vi "deleteScriptEvent.vi"(8 "error in (no error)":errorcluster, 10 "Enum":enum16{"Update_dt", "Update_Time"}(ring), 11 "ScriptEditorV2 in":refnum<class "ScriptEditorV2.lvclass">) -> (0 "error out":errorcluster, 3 "ScriptEditorV2 out":refnum<class "ScriptEditorV2.lvclass">)   [LabVIEW 2011, in "Views.lvlib" / "ScriptEditor.lvlib" / "ScriptEditorV2.lvclass"]
uses:
  ScriptEditorV2.lvclass
  ScriptEditorV2.lvclass/ScriptEditorV2.ctl
  Tools/Scripting/ScriptingEvent/ScriptEventList/ScriptEventList.lvclass
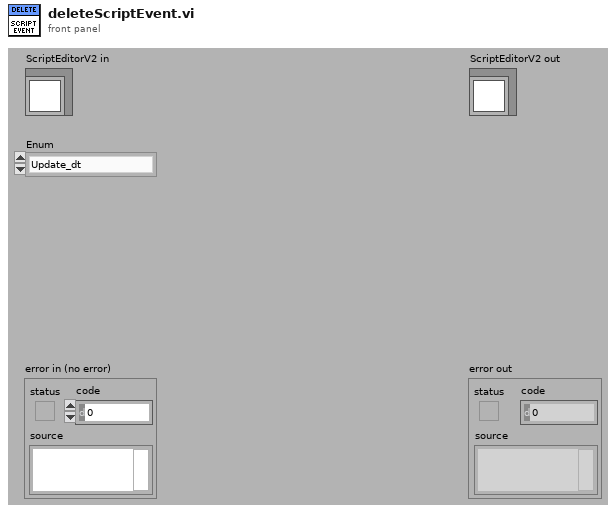
[diagram p1: front panel]
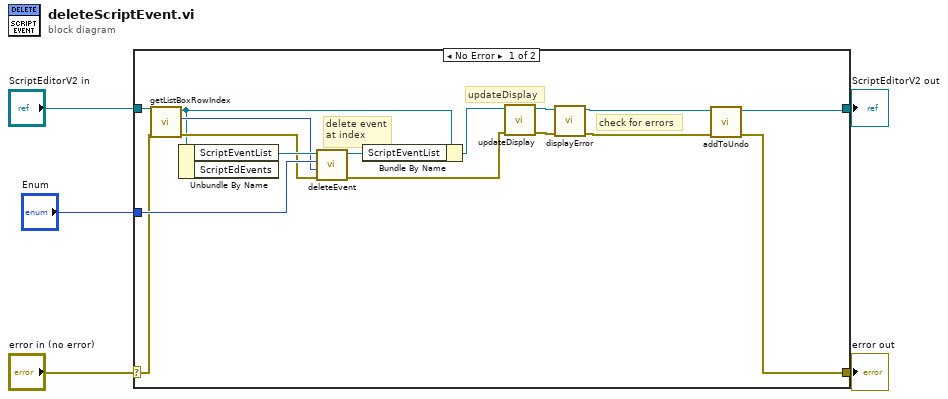
[diagram p0: block diagram]
diagram:
  n1 = case shown="No Error" "error in (no error)" {
    selector: "error in (no error)" -> [w14 w23]
    tunnel: [w6 w23] -> w4
    tunnel: [w7 w22] -> w2
    tunnel: "ScriptEditorV2 in" -> [w10 w22]
    tunnel: "Enum" -> [w20 _]
    frame No Error {
      # "delete event\nat index"
      # "check for errors"
      # "updateDisplay"
      n2 = call "getListBoxRowIndex.vi"("error in (no error)"=w14, "ScriptEditorV2 in"=w10) -> ("error out"=w13:errorcluster, "rowIndex"=w12:i32, "ScriptEditorV2 out"=w11:refnum<class "ScriptEditorV2.lvclass">)  [unwired: 7 in]
      n3 = Unbundle By Name(w11) -> ("ScriptEventList"=w21:refnum<class "ScriptEventList.lvclass">)  [unwired: 1 out]
      n4 = call "deleteEvent.vi"("error in (no error)"=w13, "selectedEvent"=w12, "Enum"=w20, "ScriptEventList in"=w21) -> ("error out"=w19:errorcluster, "ScriptEventList out"=w16:refnum<class "ScriptEventList.lvclass">)  [unwired: 6 in]
      n5 = Bundle By Name(cluster=w11, "ScriptEventList"=w16) -> (w15:refnum<class "ScriptEditorV2.lvclass">)
      n6 = call "updateDisplay.vi"("error in (no error)"=w19, "ScriptEditorV2 in"=w15) -> ("error out"=w18:errorcluster, "ScriptEditorV2 out"=w17:refnum<class "ScriptEditorV2.lvclass">)  [unwired: 8 in]
      n7 = call "displayError.vi"("error in (no error)"=w18, "ScriptEditorV2 in"=w17) -> ("error out"=w8:errorcluster, "ScriptEditorV2 out"=w9:refnum<class "ScriptEditorV2.lvclass">)  [unwired: 8 in]
      n8 = call "addToUndo.vi"("error in (no error)"=w8, "ScriptEditorV2 in"=w9) -> ("error out"=w6:errorcluster, "ScriptEditorV2 out"=w7:refnum<class "ScriptEditorV2.lvclass">)  [unwired: 8 in]
    }
    frame Error {
    }
  }
  "error out" <- w4
  "ScriptEditorV2 out" <- w2
